vi "TestInitializeOneShotSubscription_RejectOldValue.vi"(8 "error in (no error)":errorcluster, 11 "TestCase in":refnum<class "TestSubscriptionPolicy.lvclass">) -> (0 "error out":errorcluster, 3 "TestCase out":refnum<class "TestSubscriptionPolicy.lvclass">)   [LabVIEW 2017, in "TestSubscriptionPolicy.lvclass"]
uses:
  TestSubscriptionPolicy.lvclass
  OneShotSubscription/OneShotSubscription.lvclass/OneShotSubscription.ctl
  Transport/QueueTransport/QueueTransport.lvclass/QueueTransport.ctl
  IMediator/ISubscriptionPolicy/ISubscriptionPolicy.lvclass/ISubscriptionPolicy.ctl
  Transport/QueueTransport/QueueTransport.lvclass
  C:/Git/mva-framework/Framework/IMediator/ITransport/ITransport.lvclass
  OneShotSubscription/OneShotSubscription.lvclass
  C:/Git/mva-framework/Framework/IMediator/ISubscriptionPolicy/ISubscriptionPolicy.lvclass
  <vilib>/Utility/error.llb/Error Cluster From Error Code.vi
  IMediator/ISubscriptionPolicy/ISubscriptionPolicy.lvclass
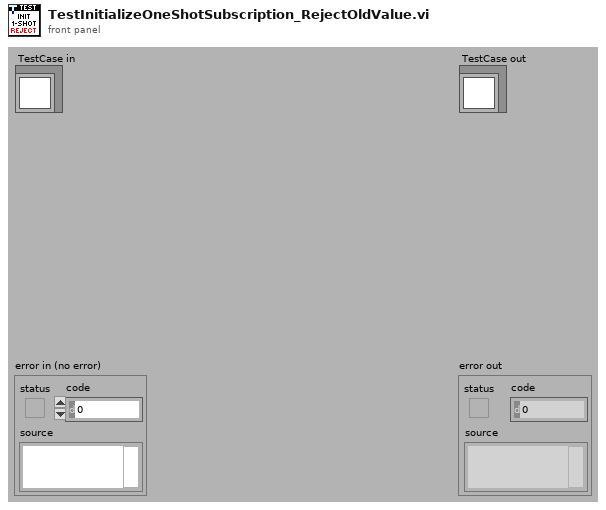
[diagram p1: front panel]
types:
  T1 = typedef "IMediator.lvlib/ISubscriptionPolicy.lvclass/ISubscriptionPolicy Reference.ctl" = refnum<data-value>
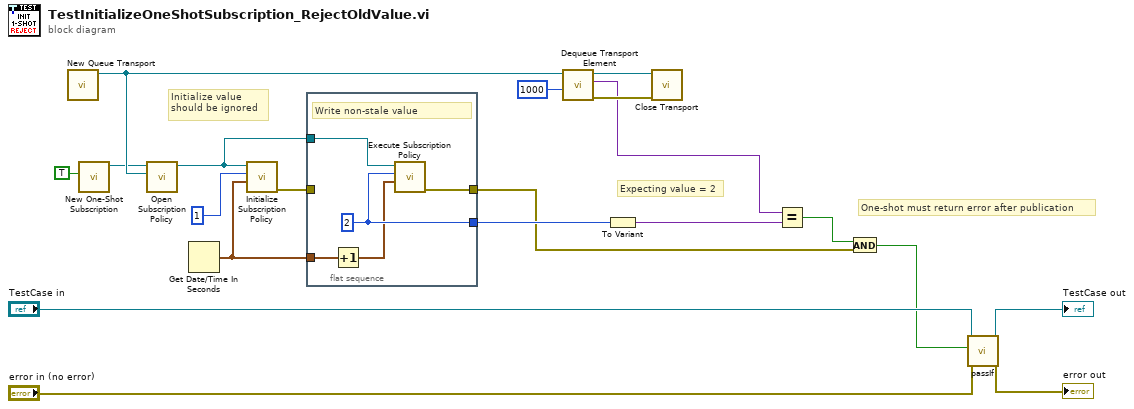
[diagram p0: block diagram]
diagram:
  # "Initialize value\nshould be ignored"
  # "One-shot must return error after publication"
  # "Expecting value = 2"
  n1 = call "New Queue Transport.vi"() -> ("QueueTransport"=w16:refnum<class "QueueTransport.lvclass">)  [unwired: 10 in, 1 out]
  n2 = call "New One-Shot Subscription.vi"("Ignore Past Updates? (F)"=TRUE) -> ("OneShotSubscription Out"=w12:refnum<class "OneShotSubscription.lvclass">)  [unwired: 10 in]
  n3 = call "Open Subscription Policy.vi"("Transport"=w16, "SubscriptionPolicy"=w12) -> ("Subscription Policy"=w5:T1)  [unwired: 8 in, 1 out]
  n4 = Get Date/Time In Seconds() -> (seconds since 1Jan1904=w3:timestamp)
  n5 = call "Initialize Subscription Policy.vi"("Last Publish Time"=w3, "Last Topic Value"=1, "Subscription Policy"=w5) -> ("Error Out (Do Not Subscribe?)"=w2:errorcluster)  [unwired: 8 in]
  n6 = flat-sequence {
    tunnel: [w25] -> w10
    tunnel: [w24] -> w7
    tunnel: w5 -> [w23]
    tunnel: w3 -> [w22]
    tunnel: w2 -> [_]
    frame #0 {
      w25 = 2
      # "Write non-stale value"
      n7 = Increment(x=w22) -> (x+1=w21:timestamp)
      n8 = call "Execute Subscription Policy.vi"("Publish Time"=w21, "New Topic Value"=w25, "Subscription Policy"=w23) -> ("error out (Unsubscribe?)"=w24:errorcluster)  [unwired: 8 in]
    }
  }
  n9 = call "Dequeue Transport Element.vi"("Timeout In ms (-1)"=1000, "QueueTransport in"=w16) -> ("error out"=w13:errorcluster, "Data"=w1:variant, "QueueTransport out"=w14:refnum<class "QueueTransport.lvclass">)  [unwired: 6 in, 1 out]
  n10 = To Variant(anything=w10) -> (Variant=w9:variant)
  n11 = call-dynamic "Close Transport.vi"("error in (no error)"=w13, "QueueTransport in"=w14) -> ()  [unwired: 9 in, 1 out]
  n12 = Equal?(x=w1, y=w9) -> (x = y?=w8:bool)
  n13 = And(x=w8, y=w7) -> (x .and. y?=w6:bool)
  n14 = call-dynamic "passIf.vi"("error in (no error)"="error in (no error)", "pass"=w6, "TestCase in"="TestCase in") -> ("error out"=→"error out":errorcluster, "TestCase out"=→"TestCase out":refnum<class "TestSubscriptionPolicy.lvclass">)  [unwired: 7 in]
